vi "Read_Out_FPGA_3Ghz.vi"(8 "Repetition Rate":bool, 9 "U8ReadFIFO":u8[](array[numeric]), 10 "U64ReadFIFO 2":u64[](array[numeric]), 11 "U64ReadFIFO1":u64[](array[numeric])) -> (2 "Trigger":bool[](array[boolean]), 3 "PMT Signal":u8[](array[numeric]))   [LabVIEW 2014]
panel:
  # "40MHz"
  # "80MHz"
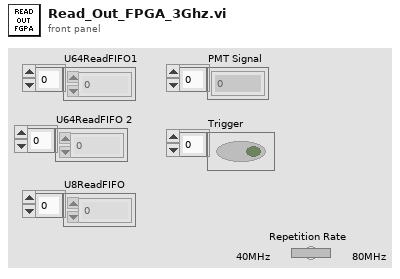
[diagram p1: front panel]
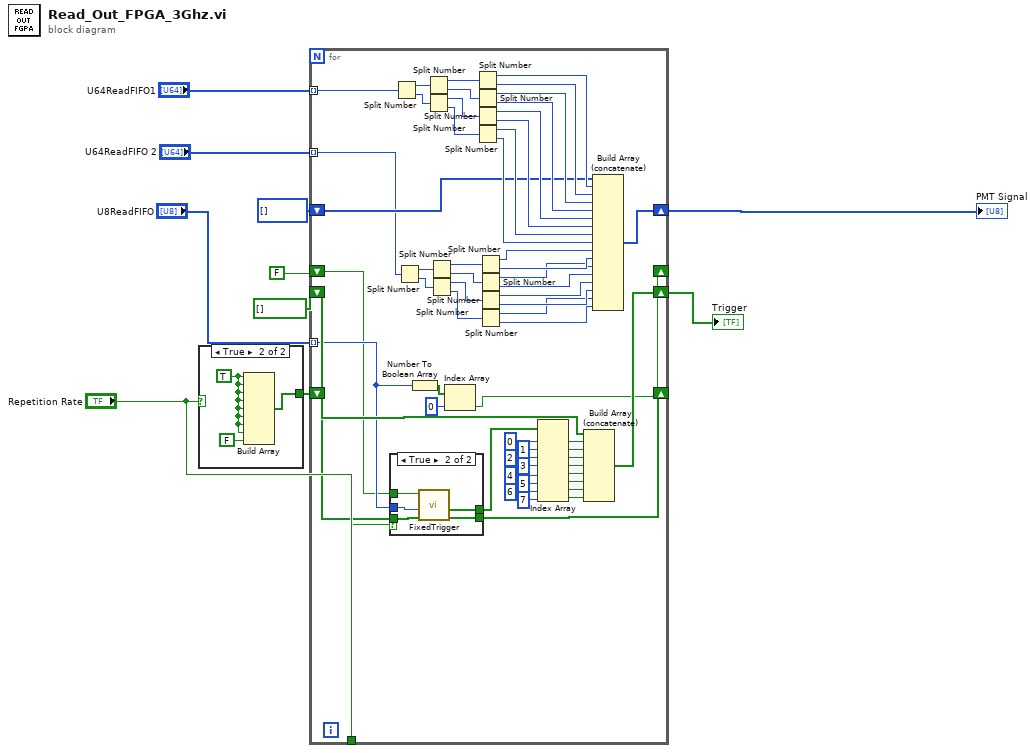
[diagram p0: block diagram]
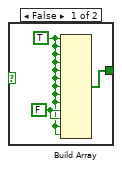
[diagram p2: hidden frame]
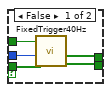
[diagram p3: hidden frame]
diagram:
  n1 = case shown="True" "Repetition Rate" {
    tunnel: [w13 w14] -> w4
    frame False {
      w12 = FALSE
      w11 = TRUE
      n2 = Build Array(w11, w11, w11, w11, w11, w11, w11, w11, w11, w12, w12, w11, w11) -> (w13:bool[])
    }
    frame True {
      w15 = TRUE
      n3 = Build Array(w15, w15, w15, w15, w15, w15, w15, w15, FALSE) -> (w14:bool[])
    }
  }
  n4 = for {
    tunnel: "U64ReadFIFO1" -> [w75] mode=indexing
    shift-right: [w60] -> w10
    shift-left: u8[] [] -> [w59]
    tunnel: "U8ReadFIFO" -> [w37] mode=indexing
    shift-right: [w58] -> w9
    shift-left: bool[] [] -> [w57]
    shift-right: [w34] -> _
    shift-left: w4 -> [w35]
    shift-right: [w38] -> _
    shift-left: FALSE -> [w36]
    tunnel: "Repetition Rate" -> [w32]
    tunnel: "U64ReadFIFO 2" -> [w25] mode=indexing
    n5 = case shown="True" w32 {
      tunnel: w37 -> [w77 w85]
      tunnel: w36 -> [w78 w84]
      tunnel: w35 -> [w76 w83]
      tunnel: [w79 w82] -> w34
      tunnel: [w80 w81] -> w33
      frame False {
        n6 = call "FixedTrigger40Hz.vi"("array in"=w76, "IO Module\\Synchronous Trigger Input"=w77, "Last? Input"=w78) -> ("array out"=w79:bool[], "trigger out"=w80:bool[])  [unwired: 7 in]
      }
      frame True {
        n7 = call "FixedTrigger.vi"("array in"=w83, "IO Module\\Synchronous Trigger Input"=w85, "Last? Input"=w84) -> ("array out"=w82:bool[], "trigger out"=w81:bool[])  [unwired: 7 in]
      }
    }
    n8 = Split Number(x=w75) -> (hi(x)=w74:u32, lo(x)=w73:u32)
    n9 = Split Number(x=w25) -> (hi(x)=w31:u32, lo(x)=w30:u32)
    n10 = Number To Boolean Array(number=w37) -> (Boolean array=w39:bool[])
    n11 = Split Number(x=w74) -> (hi(x)=w72:u16, lo(x)=w71:u16)
    n12 = Split Number(x=w73) -> (hi(x)=w70:u16, lo(x)=w69:u16)
    n13 = Split Number(x=w31) -> (hi(x)=w29:u16, lo(x)=w28:u16)
    n14 = Split Number(x=w30) -> (hi(x)=w27:u16, lo(x)=w26:u16)
    n15 = Index Array(array=w39, index=0) -> (element=w38:bool)
    n16 = Split Number(x=w72) -> (hi(x)=w68:u8, lo(x)=w67:u8)
    n17 = Split Number(x=w71) -> (hi(x)=w66:u8, lo(x)=w65:u8)
    n18 = Split Number(x=w70) -> (hi(x)=w64:u8, lo(x)=w63:u8)
    n19 = Split Number(x=w69) -> (hi(x)=w62:u8, lo(x)=w61:u8)
    n20 = Split Number(x=w29) -> (hi(x)=w24:u8, lo(x)=w23:u8)
    n21 = Split Number(x=w28) -> (hi(x)=w22:u8, lo(x)=w21:u8)
    n22 = Split Number(x=w27) -> (hi(x)=w20:u8, lo(x)=w19:u8)
    n23 = Split Number(x=w26) -> (hi(x)=w18:u8, lo(x)=w17:u8)
    n24 = Index Array(array=w33, index #1=0 ("index"), index #2=1 ("index"), index #3=2 ("index"), index #4=3 ("index"), index #5=4 ("index"), index #6=5 ("index"), index #7=6 ("index"), index #8=7 ("index")) -> (element #1=w48:bool, element #2=w47:bool, element #3=w46:bool, element #4=w45:bool, element #5=w44:bool, element #6=w43:bool, element #7=w42:bool, element #8=w41:bool)
    n25 = Build Array (concatenate)(w57, w48, w47, w46, w45, w44, w43, w42, w41) -> (w58:bool[])
    n26 = Build Array (concatenate)(w59, w68, w67, w66, w65, w64, w63, w62, w61, w24, w23, w22, w21, w20, w19, w18, w17) -> (w60:u8[])
  }
  "PMT Signal" <- w10
  "Trigger" <- w9
